vi "Deadband.vi"(10 "joystick axis":dbl format="%#_13g", 11 "DeadBand":dbl=0.15 format="%#_13g") -> (3 "Deadbanded output":dbl format="%#_13g")   [LabVIEW 2019, in "Joysticks.lvlib" / "Joysticks.lvclass"]
doc: "this VI is used to insert deadband into a joystick"
uses:
  Joysticks.lvclass
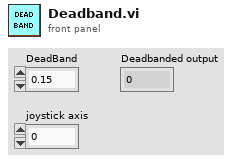
[diagram p1: front panel]
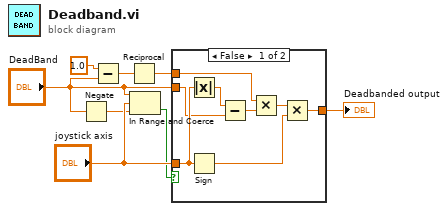
[diagram p0: block diagram]
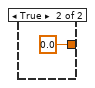
[diagram p2: hidden frame]
diagram:
  n1 = Negate(x="DeadBand") -> (-x=w3:dbl)
  n2 = Subtract(x=1.0, y="DeadBand") -> (x-y=w2:dbl)
  n3 = Reciprocal(x=w2) -> (1/x=w7:dbl)
  n4 = In Range and Coerce(upper limit="DeadBand", x="joystick axis", lower limit=w3) -> (In Range?=w4:bool)  [unwired: 1 out]
  n5 = case shown="False" w4 {
    tunnel: "joystick axis" -> [w16 _]
    tunnel: "DeadBand" -> [w12 _]
    tunnel: w7 -> [w11 _]
    tunnel: [w9 0.0] -> w8
    frame False {
      n6 = Absolute Value(x=w16) -> (abs(x)=w13:dbl)
      n7 = Sign(1:w16) -> (0:w10:dbl)
      n8 = Subtract(x=w13, y=w12) -> (x-y=w14:dbl)
      n9 = Multiply(x=w11, y=w14) -> (x*y=w15:dbl)
      n10 = Multiply(x=w15, y=w10) -> (x*y=w9:dbl)
    }
    frame True {
    }
  }
  "Deadbanded output" <- w8
